vi "Read id type.vi"(8 "error in (no error)":errorcluster, 11 "Request in":refnum<class "Request.lvclass">) -> (0 "error out":errorcluster, 2 "type":enum16{"none", "String", "Number", "NULL"}(ring), 3 "Request out":refnum<class "Request.lvclass">)   [LabVIEW 2015]
uses:
  id/id.lvclass
  Request.lvclass
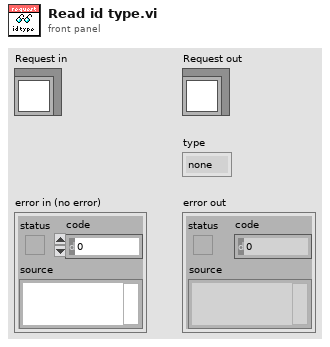
[diagram p1: front panel]
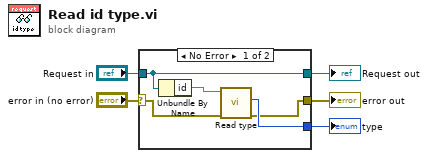
[diagram p0: block diagram]
diagram:
  n1 = case shown="No Error" "error in (no error)" {
    selector: "error in (no error)" -> [w6 w11]
    tunnel: [w7 w11] -> w4
    tunnel: [w10 w12] -> w2
    tunnel: "Request in" -> [w10 w12]
    tunnel: [w8 _] -> w1
    frame No Error {
      n2 = Unbundle By Name(w10) -> ("id"=w9)
      n3 = call-dynamic "Read type.vi"("error in (no error)"=w6, "id in"=w9) -> ("error out"=w7:errorcluster, "type"=w8:enum16{"none", "String", "Number", "NULL"})  [unwired: 7 in, 1 out]
    }
    frame Error {
    }
  }
  "error out" <- w4
  "Request out" <- w2
  "type" <- w1
